vi "writeControlDataToString_v04.vi"(11 "Ctl Refnum":refnum<vi>) -> (3 "String written to file":string)   [LabVIEW 2019]
uses:
  <vilib>/Utility/Data Type/NI_Data Type.lvlib
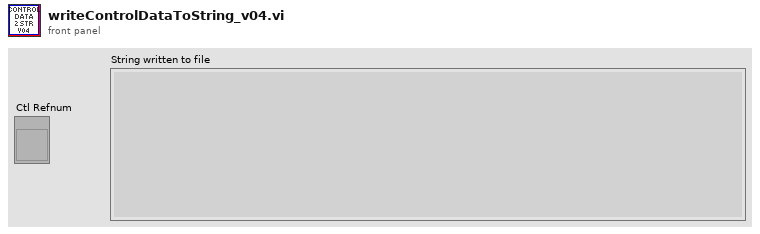
[diagram p1: front panel]
types:
  T1 = typedef "NI_Data Type.lvlib/Data Type.ctl" = enum8{"Invalid Type", "Void", "I8", "I16", "I32", "I64", "U8", "U16", "U32", "U64", "Single Float", "Double Float", "Extended Float", "Single Complex", "Double Complex", "Extended Complex", "Enum U8", "Enum U16", "Enum U32", "Enum U64", "Single Float With Unit", "Double Float With Unit", "Extended Float With Unit", "Single Complex with Unit", "Double Complex with Unit", "Extended Complex with Unit", "Boolean", "String", "Path", "Picture", "Tag", "Array", "Cluster", "Variant", "LV Variant", "Waveform", "Timestamp", "Digital Waveform", "Digital Data", "ExpressData", "Refnum", "External Data", "VI", "Poly VI", "LabVIEW Class Instance", "Fixed Point", "Set Collection", "Map Collection"}
  T2 = typedef "NI_Data Type.lvlib/Type Definition Info.ctl" = cluster{"Name":string, "Timestamp":u32}
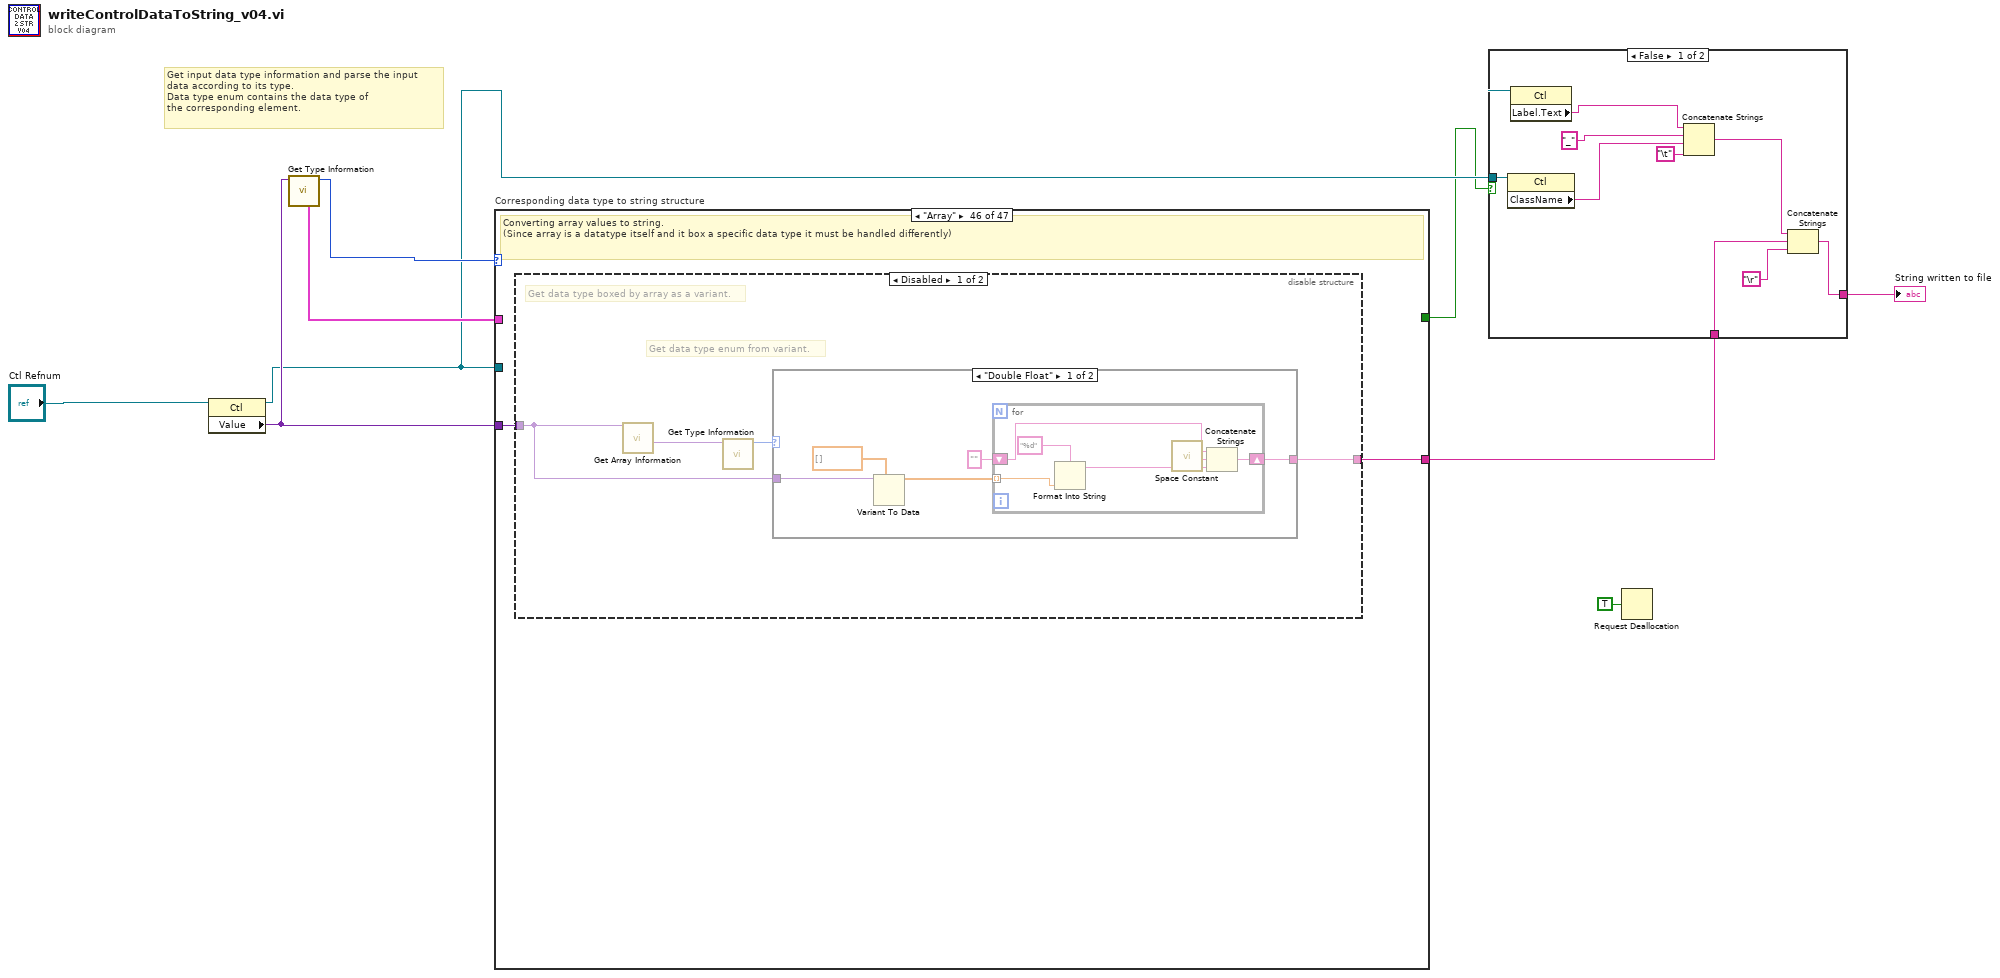
[diagram p0: block diagram]
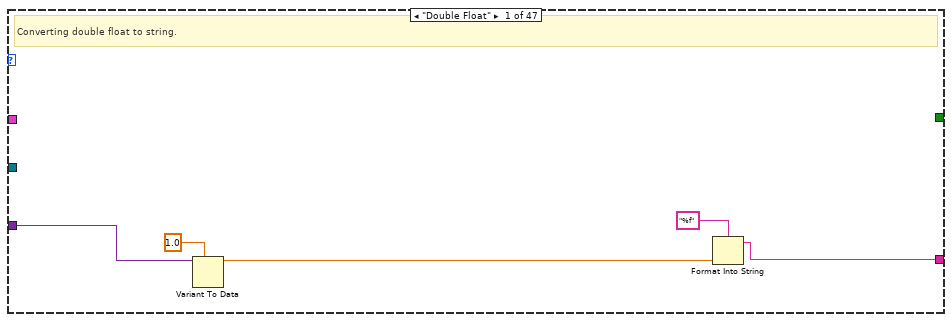
[diagram p3: hidden frame]
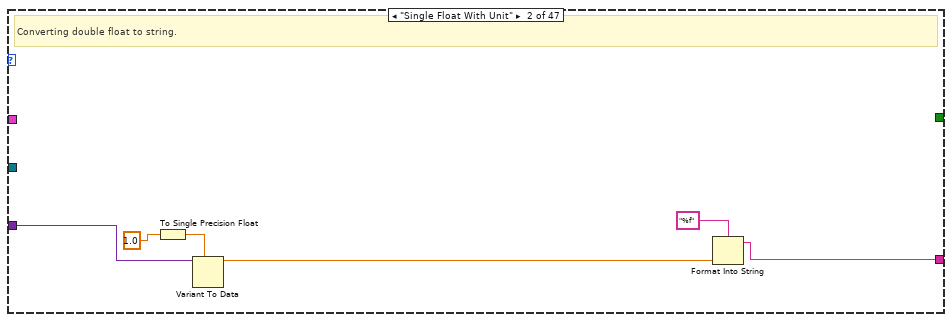
[diagram p4: hidden frame]
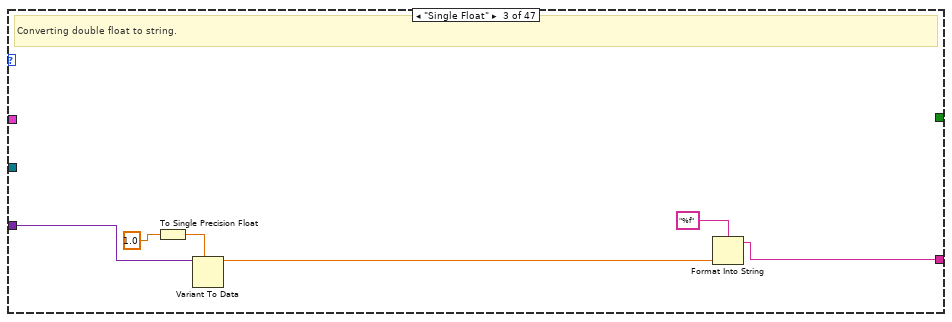
[diagram p5: hidden frame]
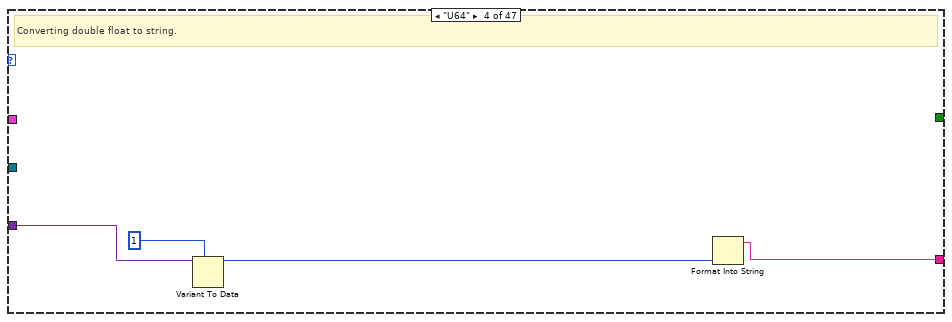
[diagram p6: hidden frame]
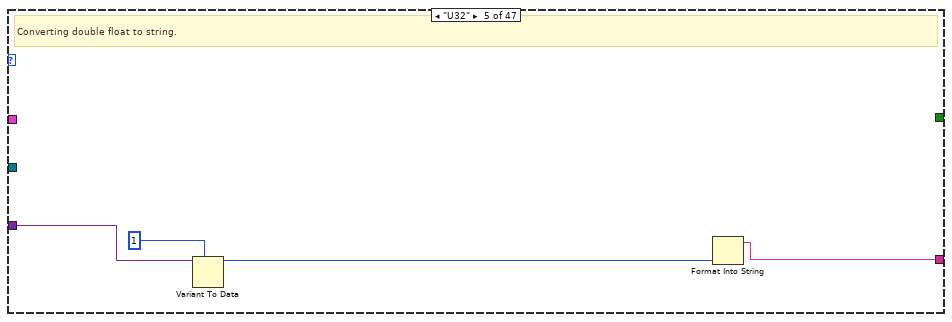
[diagram p7: hidden frame]
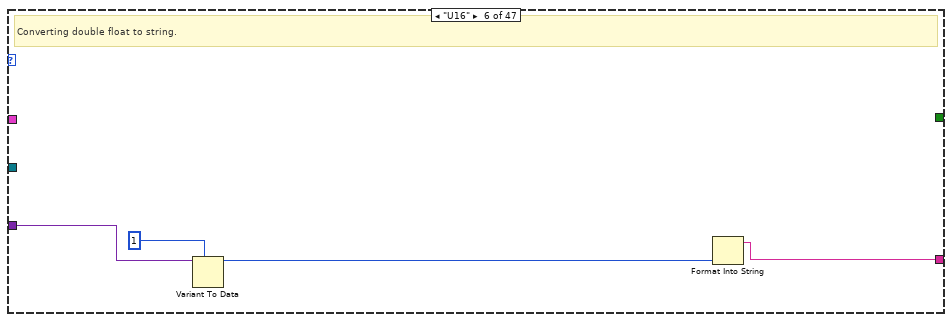
[diagram p8: hidden frame]
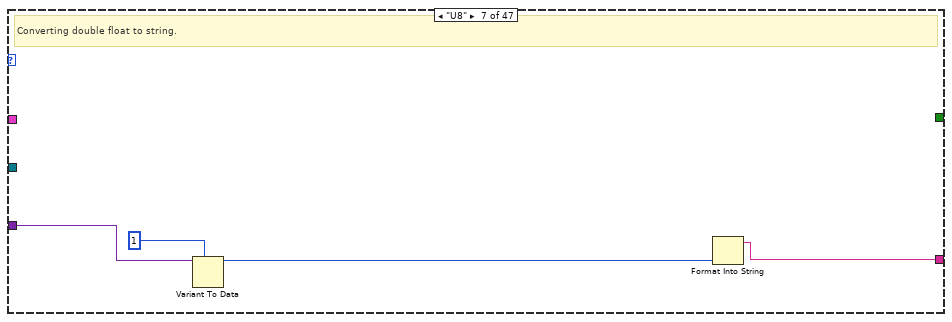
[diagram p9: hidden frame]
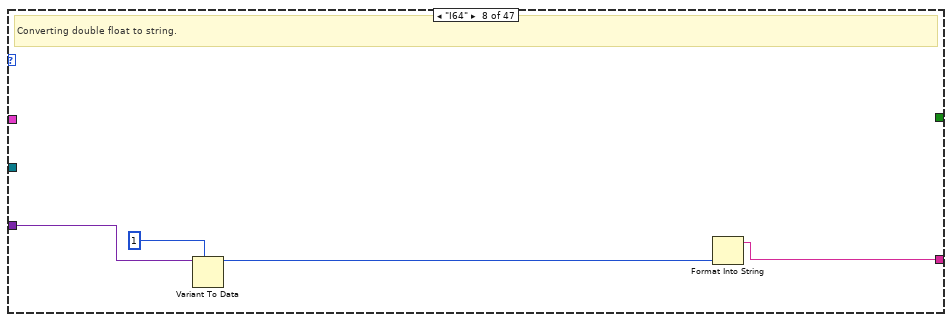
[diagram p10: hidden frame]
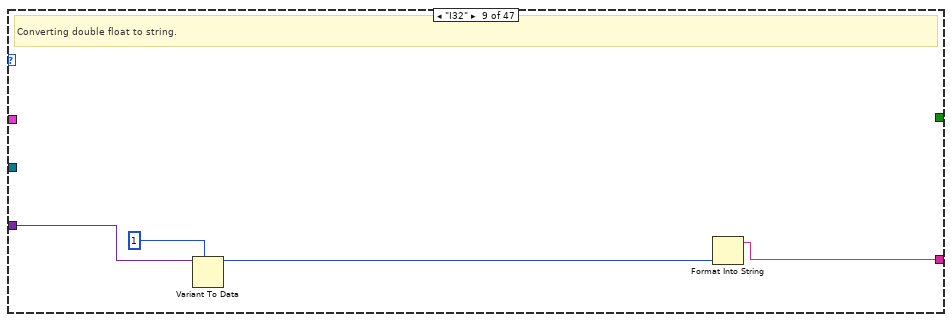
[diagram p11: hidden frame]
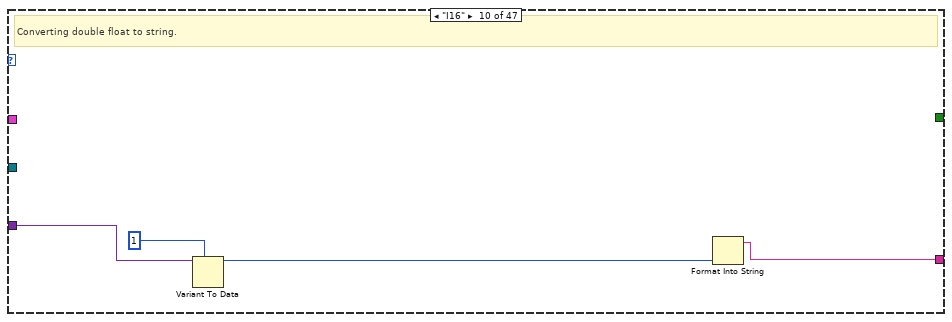
[diagram p12: hidden frame]
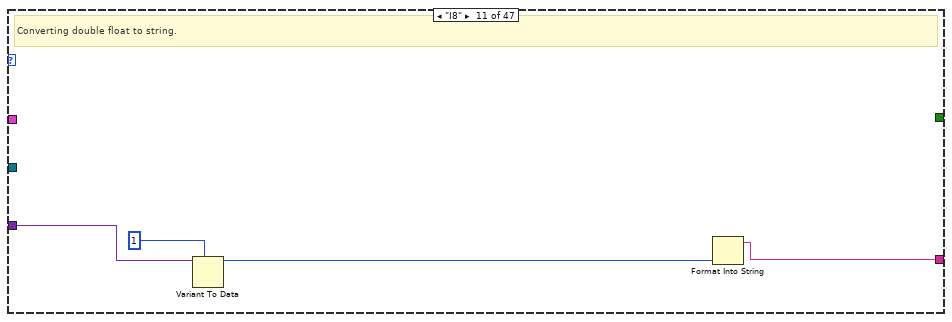
[diagram p13: hidden frame]
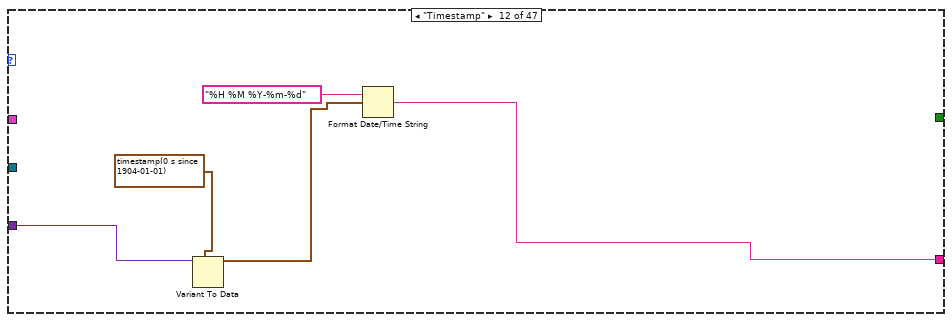
[diagram p14: hidden frame]
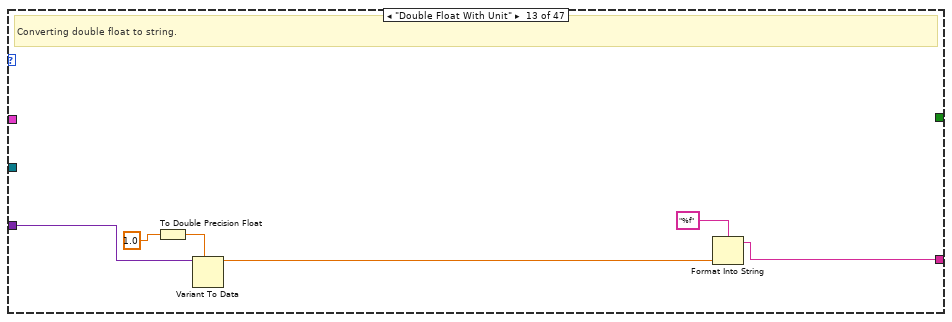
[diagram p15: hidden frame]
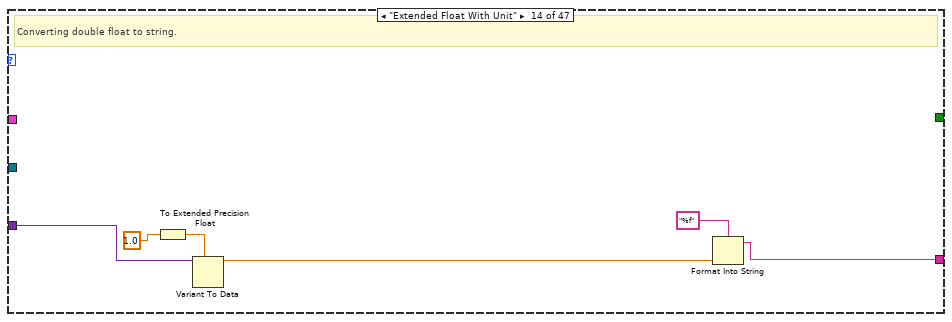
[diagram p16: hidden frame]
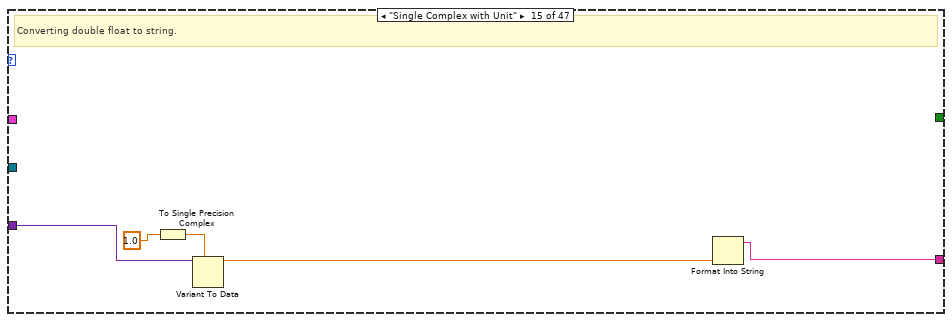
[diagram p17: hidden frame]
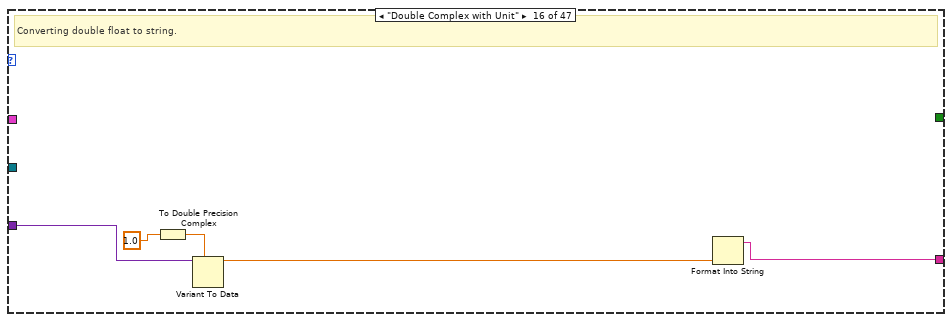
[diagram p18: hidden frame]
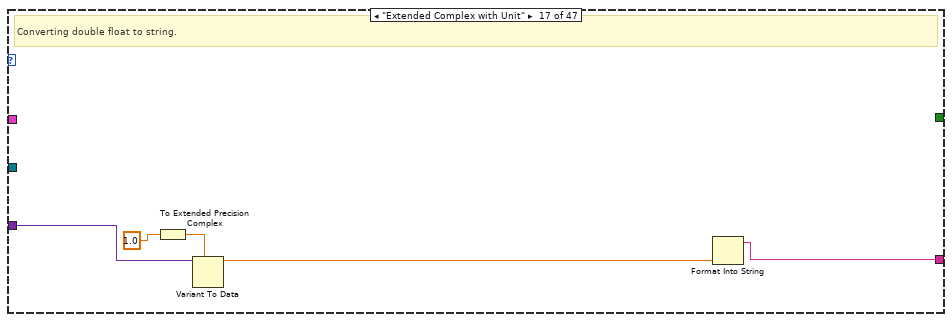
[diagram p19: hidden frame]
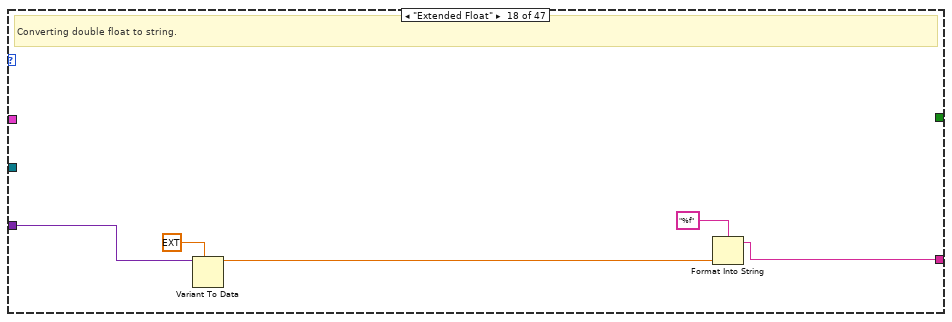
[diagram p20: hidden frame]
diagram:
  # "Get input data type information and parse the input \ndata according to its type.\nData type enum contains the data type of \nthe corresponding element."
  n1 = property class="Ctl"(reference="Ctl Refnum") -> (reference out=w5:refnum<vi>, "Value"=w8:variant)  [unwired: 1 in, 1 out]
  n2 = call <vilib>:"Get Type Information.vi"("variant"=w8) -> ("type"=w9:T1, "type definition info"=w6:T2)  [unwired: 6 in, 3 out]
  n3 = case "Corresponding data type to string structure" shown="\"Array\"" w9 {
    tunnel: w8 -> [w10 w17 w23 w28 w32 w36 w40 w44 w48 w52 w56 w63 w66 w72 w78 w83 w88 w91 w96 w100 w104 _ _ _ _ _ _ _ _ _ _ _ _ _ _ _ _ _ _ _ _ _ _ w200 w203 w205 _]
    tunnel: [w13 w20 w26 w30 w34 w38 w42 w46 w50 w54 w58 w59 w69 w75 w80 w85 w90 w94 w98 w102 w106 w109 w116 w122 w131 w135 w142 w149 w154 "NA" ("Label.Text") "NA" ("Label.Text") "NA" ("Label.Text") "NA" ("Label.Text") "NA" ("Label.Text") "NA" ("Label.Text") "NA" ("Label.Text") "NA" ("Label.Text") "NA" ("Label.Text") w180 "NA" ("Label.Text") "NA" ("Label.Text") "NA" ("Label.Text") "NA" ("Label.Text") w195 w201 w204 w224] -> w4
    tunnel: w5 -> [_ _ _ _ _ _ _ _ _ _ _ _ _ _ _ _ _ _ _ _ _ w114 w121 w123 w134 w141 w148 w153 w157 _ _ _ _ _ _ _ _ _ w170 _ _ _ _ _ _ _ _]
    tunnel: w6 -> [_ _ _ _ _ _ _ _ _ _ _ _ _ _ _ _ _ _ _ _ _ _ _ _ _ _ _ _ _ _ _ _ _ _ _ _ _ _ _ _ _ _ _ _ _ _ w223]
    tunnel: [_ _ _ _ _ _ _ _ _ _ _ _ _ _ _ _ _ _ _ _ _ _ _ _ _ _ _ _ _ _ _ FALSE _ _ _ _ _ _ _ _ _ _ _ _ _ _ _] -> w2
    frame "Double Float" {
      # "Converting double float to string."
      n4 = Variant To Data(type=1.0 ("Age"), Variant=w10) -> (data=w11:dbl)  [unwired: 1 in, 1 out]
      n5 = Format Into String(format string="%f", w11) -> (resulting string=w13:string)  [unwired: 2 in, 1 out]
    }
    frame "Single Float With Unit" {
      # "Converting double float to string."
      n6 = To Single Precision Float(number=1.0 ("Age")) -> (single precision float=w15:sgl)
      n7 = Variant To Data(type=w15, Variant=w17) -> (data=w18:sgl)  [unwired: 1 in, 1 out]
      n8 = Format Into String(format string="%f", w18) -> (resulting string=w20:string)  [unwired: 2 in, 1 out]
    }
    frame "Single Float" {
      # "Converting double float to string."
      n9 = To Single Precision Float(number=1.0 ("Age")) -> (single precision float=w21:sgl)
      n10 = Variant To Data(type=w21, Variant=w23) -> (data=w24:sgl)  [unwired: 1 in, 1 out]
      n11 = Format Into String(format string="%f", w24) -> (resulting string=w26:string)  [unwired: 2 in, 1 out]
    }
    frame "U64" {
      # "Converting double float to string."
      n12 = Variant To Data(type=u64 1 ("Age"), Variant=w28) -> (data=w29:u64)  [unwired: 1 in, 1 out]
      n13 = Format Into String(w29) -> (resulting string=w30:string)  [unwired: 3 in, 1 out]
    }
    frame "U32" {
      # "Converting double float to string."
      n14 = Variant To Data(type=u32 1 ("Age"), Variant=w32) -> (data=w33:u32)  [unwired: 1 in, 1 out]
      n15 = Format Into String(w33) -> (resulting string=w34:string)  [unwired: 3 in, 1 out]
    }
    frame "U16" {
      # "Converting double float to string."
      n16 = Variant To Data(type=u16 1 ("Age"), Variant=w36) -> (data=w37:u16)  [unwired: 1 in, 1 out]
      n17 = Format Into String(w37) -> (resulting string=w38:string)  [unwired: 3 in, 1 out]
    }
    frame "U8" {
      # "Converting double float to string."
      n18 = Variant To Data(type=u8 1 ("Age"), Variant=w40) -> (data=w41:u8)  [unwired: 1 in, 1 out]
      n19 = Format Into String(w41) -> (resulting string=w42:string)  [unwired: 3 in, 1 out]
    }
    frame "I64" {
      # "Converting double float to string."
      n20 = Variant To Data(type=i64 1 ("Age"), Variant=w44) -> (data=w45:i64)  [unwired: 1 in, 1 out]
      n21 = Format Into String(w45) -> (resulting string=w46:string)  [unwired: 3 in, 1 out]
    }
    frame "I32" {
      # "Converting double float to string."
      n22 = Variant To Data(type=1 ("Age"), Variant=w48) -> (data=w49:i32)  [unwired: 1 in, 1 out]
      n23 = Format Into String(w49) -> (resulting string=w50:string)  [unwired: 3 in, 1 out]
    }
    frame "I16" {
      # "Converting double float to string."
      n24 = Variant To Data(type=i16 1 ("Age"), Variant=w52) -> (data=w53:i16)  [unwired: 1 in, 1 out]
      n25 = Format Into String(w53) -> (resulting string=w54:string)  [unwired: 3 in, 1 out]
    }
    frame "I8" {
      # "Converting double float to string."
      n26 = Variant To Data(type=i8 1 ("Age"), Variant=w56) -> (data=w57:i8)  [unwired: 1 in, 1 out]
      n27 = Format Into String(w57) -> (resulting string=w58:string)  [unwired: 3 in, 1 out]
    }
    frame "Timestamp" {
      n28 = Variant To Data(type=timestamp(0 s since 1904-01-01), Variant=w63) -> (data=w60:timestamp)  [unwired: 1 in, 1 out]
      n29 = Format Date/Time String(time format string (%c)="%H %M %Y-%m-%d", seconds (now)=w60) -> (date/time string=w59:string)  [unwired: 1 in]
    }
    frame "Double Float With Unit" {
      # "Converting double float to string."
      n30 = To Double Precision Float(number=1.0 ("Age")) -> (double precision float=w64:dbl)
      n31 = Variant To Data(type=w64, Variant=w66) -> (data=w67:dbl)  [unwired: 1 in, 1 out]
      n32 = Format Into String(format string="%f", w67) -> (resulting string=w69:string)  [unwired: 2 in, 1 out]
    }
    frame "Extended Float With Unit" {
      # "Converting double float to string."
      n33 = To Extended Precision Float(1:1.0 ("Age")) -> (0:w70:ext)
      n34 = Variant To Data(type=w70, Variant=w72) -> (data=w73:ext)  [unwired: 1 in, 1 out]
      n35 = Format Into String(format string="%f", w73) -> (resulting string=w75:string)  [unwired: 2 in, 1 out]
    }
    frame "Single Complex with Unit" {
      # "Converting double float to string."
      n36 = To Single Precision Complex(1:1.0 ("Age")) -> (0:w76:csg)
      n37 = Variant To Data(type=w76, Variant=w78) -> (data=w79:csg)  [unwired: 1 in, 1 out]
      n38 = Format Into String(w79) -> (resulting string=w80:string)  [unwired: 3 in, 1 out]
    }
    frame "Double Complex with Unit" {
      # "Converting double float to string."
      n39 = To Double Precision Complex(1:1.0 ("Age")) -> (0:w81:cdb)
      n40 = Variant To Data(type=w81, Variant=w83) -> (data=w84:cdb)  [unwired: 1 in, 1 out]
      n41 = Format Into String(w84) -> (resulting string=w85:string)  [unwired: 3 in, 1 out]
    }
    frame "Extended Complex with Unit" {
      # "Converting double float to string."
      n42 = To Extended Precision Complex(1:1.0 ("Age")) -> (0:w86:cxt)
      n43 = Variant To Data(type=w86, Variant=w88) -> (data=w89:cxt)  [unwired: 1 in, 1 out]
      n44 = Format Into String(w89) -> (resulting string=w90:string)  [unwired: 3 in, 1 out]
    }
    frame "Extended Float" {
      # "Converting double float to string."
      n45 = Variant To Data(type=ext 1.0 ("Age"), Variant=w91) -> (data=w92:ext)  [unwired: 1 in, 1 out]
      n46 = Format Into String(format string="%f", w92) -> (resulting string=w94:string)  [unwired: 2 in, 1 out]
    }
    frame "Single Complex" {
      # "Converting double float to string."
      n47 = Variant To Data(type=csg 1.0+0.0i ("Age"), Variant=w96) -> (data=w97:csg)  [unwired: 1 in, 1 out]
      n48 = Format Into String(w97) -> (resulting string=w98:string)  [unwired: 3 in, 1 out]
    }
    frame "Double Complex" {
      # "Converting double float to string."
      n49 = Variant To Data(type=cdb 1.0+0.0i ("Age"), Variant=w100) -> (data=w101:cdb)  [unwired: 1 in, 1 out]
      n50 = Format Into String(w101) -> (resulting string=w102:string)  [unwired: 3 in, 1 out]
    }
    frame "Extended Complex" {
      # "Converting double float to string."
      n51 = Variant To Data(type=cxt 1.0+0.0i ("Age"), Variant=w104) -> (data=w105:cxt)  [unwired: 1 in, 1 out]
      n52 = Format Into String(w105) -> (resulting string=w106:string)  [unwired: 3 in, 1 out]
    }
    frame "Enum U8" {
      w113 = refnum<vi> refnum  # Enum
      n53 = To More Specific Class(target class=w113, reference=w114) -> (specific class reference=w108:refnum<vi>)  [unwired: 1 in, 1 out]
      n54 = property class="Enum"(reference=w108) -> ("Strings []"=w112:string[])  [unwired: 1 in, 2 out]
      n55 = property class="Enum"(reference=w108) -> ("DigDisp.Text"=w111:string)  [unwired: 1 in, 2 out]
      n56 = Decimal String To Number(string=w111) -> (number=w110:i32)  [unwired: 2 in, 1 out]
      n57 = Index Array(array=w112, index=w110) -> (element=w109:string)
    }
    frame "Enum U16" {
      w120 = refnum<vi> refnum  # Enum
      # "Converting double float to string."
      n58 = To More Specific Class(target class=w120, reference=w121) -> (specific class reference=w115:refnum<vi>)  [unwired: 1 in, 1 out]
      n59 = property class="Enum"(reference=w115) -> ("Strings []"=w119:string[])  [unwired: 1 in, 2 out]
      n60 = property class="Enum"(reference=w115) -> ("DigDisp.Text"=w118:string)  [unwired: 1 in, 2 out]
      n61 = Decimal String To Number(string=w118) -> (number=w117:i32)  [unwired: 2 in, 1 out]
      n62 = Index Array(array=w119, index=w117) -> (element=w116:string)
    }
    frame "Enum U32" {
      # "Converting double float to string."
      n63 = disable-structure shown="Disabled" {
        disable-tunnel: w123 -> [w130 _]
        disable-tunnel: [w124 _] -> w122
        frame Disabled {
          w129 = refnum<vi> refnum  # Enum
          n64 = To More Specific Class(target class=w129, reference=w130) -> (specific class reference=w125:refnum<vi>)  [unwired: 1 in, 1 out]
          n65 = property class="Enum"(reference=w125) -> ("Strings []"=w128:string[])  [unwired: 1 in, 2 out]
          n66 = property class="Enum"(reference=w125) -> ("DigDisp.Text"=w127:string)  [unwired: 1 in, 2 out]
          n67 = Decimal String To Number(string=w127) -> (number=w126:i32)  [unwired: 2 in, 1 out]
          n68 = Index Array(array=w128, index=w126) -> (element=w124:string)
        }
        frame Enabled {
        }
      }
    }
    frame "Digital Data" {
      w133 = refnum<vi> refnum  # Digital
      # "Converting double float to string."
      n69 = To More Specific Class(target class=w133, reference=w134) -> (specific class reference=w132:refnum<vi>)  [unwired: 1 in, 1 out]
      n70 = property class="DigNum"(reference=w132) -> ("NumText.Text"=w131:string)  [unwired: 1 in, 2 out]
    }
    frame "Fixed Point" {
      w140 = refnum<vi> refnum  # Numeric
      # "Converting double float to string."
      n71 = To More Specific Class(target class=w140, reference=w141) -> (specific class reference=w139:refnum<vi>)  [unwired: 1 in, 1 out]
      n72 = property class="Num"(reference=w139) -> ("Value"=w138:variant)  [unwired: 1 in, 2 out]
      n73 = Variant To Data(type=0, Variant=w138) -> (data=w136:i32)  [unwired: 1 in, 1 out]
      n74 = Number To Decimal String(number=w136) -> (decimal integer string=w135:string)  [unwired: 1 in]
    }
    frame "Enum U64" {
      w147 = refnum<vi> refnum  # Enum
      # "Converting double float to string."
      n75 = To More Specific Class(target class=w147, reference=w148) -> (specific class reference=w143:refnum<vi>)  [unwired: 1 in, 1 out]
      n76 = property class="Enum"(reference=w143) -> ("Strings []"=w146:string[])  [unwired: 1 in, 2 out]
      n77 = property class="Enum"(reference=w143) -> ("DigDisp.Text"=w145:string)  [unwired: 1 in, 2 out]
      n78 = Decimal String To Number(string=w145) -> (number=w144:i32)  [unwired: 2 in, 1 out]
      n79 = Index Array(array=w146, index=w144) -> (element=w142:string)
    }
    frame "Path" {
      w152 = refnum<vi> refnum  # Path
      # "Converting double float to string."
      n80 = To More Specific Class(target class=w152, reference=w153) -> (specific class reference=w151:refnum<vi>)  [unwired: 1 in, 1 out]
      n81 = property class="Path"(reference=w151) -> ("Value"=w150:path)  [unwired: 1 in, 2 out]
      n82 = Path To String(path=w150) -> (string=w149:string)
    }
    frame "Picture" {
      w156 = refnum<vi> refnum  # Picture
      # "maybe save file and write path?"
      # "Converting double float to string."
      n83 = To More Specific Class(target class=w156, reference=w157) -> (specific class reference=w155:refnum<vi>)  [unwired: 1 in, 1 out]
      n84 = property class="Pict"(reference=w155) -> ("Label.Text"=w154:string)  [unwired: 1 in, 2 out]
    }
    frame "Tag" {
      # "Converting double float to string."
    }
    frame "ExpressData" {
      # "Converting double float to string."
    }
    frame "Refnum" {
      # "Converting double float to string."
    }
    frame "External Data" {
      # "Converting double float to string."
    }
    frame "VI" {
      # "Converting double float to string."
    }
    frame "Void" {
      # "Converting double float to string."
    }
    frame "Invalid Type" {
      # "Converting double float to string."
    }
    frame "Poly VI" {
      # "Converting double float to string."
    }
    frame "LabVIEW Class Instance" {
      # "Converting double float to string."
    }
    frame "Cluster" {
      w175 = "\r" ("string")
      w185 = refnum<vi> refnum  # Cluster
      n85 = To More Specific Class(target class=w185, reference=w170) -> (specific class reference=w183:refnum<vi>)  [unwired: 1 in, 1 out]
      n86 = property class="Clust"(reference=w183) -> ("AllObjs[]"=w184:refnum<vi>[])  [unwired: 1 in, 2 out]
      n87 = property class="Clust"(reference=w183) -> ("Controls[]"=w182:refnum<vi>[])  [unwired: 1 in, 2 out]
      n88 = for {
        N -> [w186]
        shift-right: [w190] -> w181
        shift-left: "" -> [w189]
        tunnel: w182 -> [w188] mode=indexing
        tunnel: w184 -> [_] mode=indexing
        tunnel: [w186] -> w178
        n89 = call "writeControlDataToString_v04.vi"("Ctl Refnum"=w188) -> ("String written to file"=w187:string)  [unwired: 10 in]
        n90 = Concatenate Strings(w189, w187) -> (w190:string)
      }
      n91 = property class="Ctl"(reference=w170) -> ("ClassName"=w171:string)  [unwired: 1 in, 2 out]
      n92 = property class="Ctl"(reference=w170) -> ("Label.Text"=w172:string)  [unwired: 1 in, 2 out]
      n93 = Concatenate Strings(w172, "_" ("string"), w171, "\t", "End" ("string")) -> (w168:string)
      n94 = Number To Decimal String(number=w178) -> (decimal integer string=w177:string)  [unwired: 1 in]
      n95 = Concatenate Strings("\t", w177, w175, w181, w168, w175) -> (w180:string)
    }
    frame "Variant" {
    }
    frame "LV Variant" {
    }
    frame "Waveform" {
    }
    frame "Digital Waveform" {
    }
    frame "Boolean" {
      # "Converting boolean float to string."
      n96 = Variant To Data(type=FALSE ("Boolean"), Variant=w200) -> (data=w198:bool)  [unwired: 1 in, 1 out]
      n97 = Select(t="True", s=w198, f="False") -> (s? t:f=w195:string)
    }
    frame "String" {
      # "Converting string to string is not required."
      n98 = Variant To Data(type="", Variant=w203) -> (data=w201:string)  [unwired: 1 in, 1 out]
    }
    frame "Array" {
      # "Converting array values to string.\n(Since array is a datatype itself and it box a specific data type it must be handled differently)"
      n99 = disable-structure shown="Disabled" {
        disable-tunnel: w205 -> [w209 _]
        disable-tunnel: [w207 _] -> w204
        frame Disabled {
          # "Get data type enum from variant."
          # "Get data type boxed by array as a variant."
          n100 = call <vilib>:"Get Array Information.vi"("variant"=w209) -> ("array element data type"=w206:variant)  [unwired: 7 in, 3 out]
          n101 = call <vilib>:"Get Type Information.vi"("variant"=w206) -> ("type"=w208:T1)  [unwired: 6 in, 4 out]
          n102 = case shown="\"Double Float\"" w208 {
            tunnel: w209 -> [w214 _]
            tunnel: [w210 "Data is not parsed"] -> w207
            frame "Double Float" {
              n103 = Variant To Data(type=dbl[] [], Variant=w214) -> (data=w212:dbl[])  [unwired: 1 in, 1 out]
              n104 = for {
                tunnel: w212 -> [w220] mode=indexing
                shift-right: [w218] -> w210
                shift-left: "" -> [w216]
                n105 = Format Into String "Format Into String"(format string="%d", w220) -> (resulting string=w217:string)  [unwired: 2 in, 1 out]
                n106 = call <vilib>:"Space Constant.vi"() -> ("String"=w215:string)
                n107 = Concatenate Strings(w216, w215, w217) -> (w218:string)
              }
            }
            frame Default {
              # "Unhandled cases."
            }
          }
        }
        frame Enabled {
        }
      }
    }
    frame Default {
      # "Unhandled datatypes."
      n108 = Unbundle By Name(w223) -> ("Name"=w222:string)
      n109 = Concatenate Strings("Data is not parsed : ", w222) -> (w224:string)
    }
  }
  n110 = case shown="False" w2 {
    tunnel: w5 -> [w234 _]
    tunnel: w4 -> [w232 w235]
    tunnel: [w230 w235] -> w3
    frame False {
      n111 = property class="Ctl"(reference=w234) -> ("ClassName"=w226:string)  [unwired: 1 in, 2 out]
      n112 = property class="Ctl"(reference=w234) -> ("Label.Text"=w227:string)  [unwired: 1 in, 2 out]
      n113 = Concatenate Strings(w227, "_" ("string"), w226, "\t") -> (w233:string)
      n114 = Concatenate Strings(w233, w232, "\r" ("string")) -> (w230:string)
    }
    frame True {
    }
  }
  "String written to file" <- w3
  n115 = Request Deallocation(TRUE ("flag")) -> ()
